vi "Rotation to Encoder Ticks.vi"(7 "Clockwise?":bool=TRUE, 11 "Degrees":dbl format="%#_13g") -> (3 "Difference in Ticks":dbl format="%#_13g")   [LabVIEW 2016]
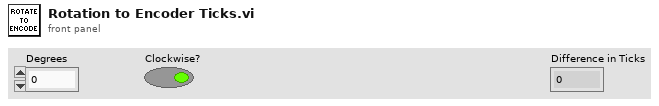
[diagram p1: front panel]
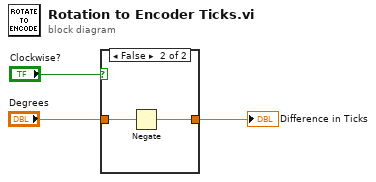
[diagram p0: block diagram]
diagram:
  n1 = case shown="False" "Clockwise?" {
    tunnel: "Degrees" -> [w4 w6]
    tunnel: [w4 w5] -> w1
    frame True {
    }
    frame False {
      n2 = Negate(x=w6) -> (-x=w5:dbl)
    }
  }
  "Difference in Ticks" <- w1
